vi "JLINKARM Exec Command.vi"(8 "error in (no error)":errorcluster, 9 "BufferSize":i32, 10 "pOut":string, 11 "pIn":string) -> (0 "error out":errorcluster, 2 "pOut out":string, 3 "function return":i32)   [LabVIEW 2020, in "JLinkARM.lvlib"]
doc: "JLINKARMDLL_API int JLINKARM_ExecCommand (const char* pIn, char* pOut, int BufferSize);"
uses:
  Lib/JLinkARM.lvlib
  JLinkARM.dll
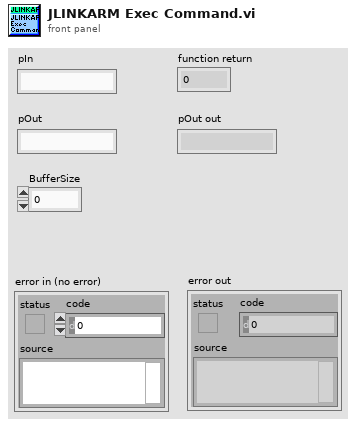
[diagram p1: front panel]
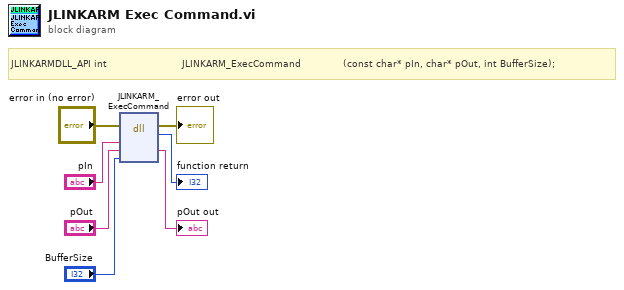
[diagram p0: block diagram]
diagram:
  # "JLINKARMDLL_API int                         JLINKARM_ExecCommand              (const char* pIn, char* pOut, int BufferSize);"
  n1 = dll-call lib="C:/Users/anybody/Desktop/JLinkARM.*" fn="JLINKARM_ExecCommand"(error in="error in (no error)", "pIn"="pIn", "pOut"="pOut", "BufferSize"="BufferSize") -> (error out=→"error out":errorcluster, →"function return":i32, "pOut"=→"pOut out":string)  [unwired: 4 in, 1 out]
